vi "Configure Trigger.vi"(6 "Validation Channel (0: A)":i32(ring) items=["A", "B", "A/B"], 7 "Trigger Mode (0: mttAuto)":i32(ring) items=["mttAuto", "mttTrigger", "mttValLoose", "mttValNorm", "mttValTight"], 8 "error in (no error)":errorcluster, 9 "Trigger Delay (0 s)":dbl, 10 "Analyzer (0: A0)":i32(ring) items=["A0", "A1"], 11 "VISA resource name":refnum<visa-resource-name>) -> (0 "error out":errorcluster, 3 "VISA resource name out":refnum<visa-resource-name>)   [LabVIEW 2014, in "Stanford Research SR1.lvlib"]
doc: "Configures the attributes for the Trigger."
uses:
  Stanford Research SR1.lvlib
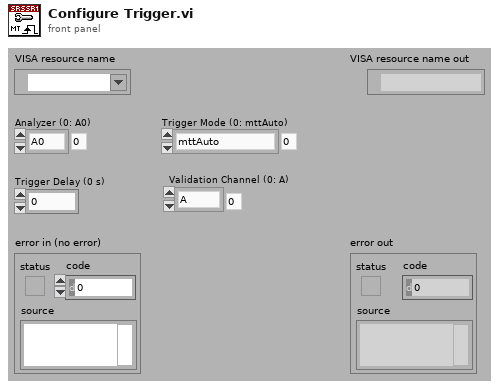
[diagram p1: front panel]
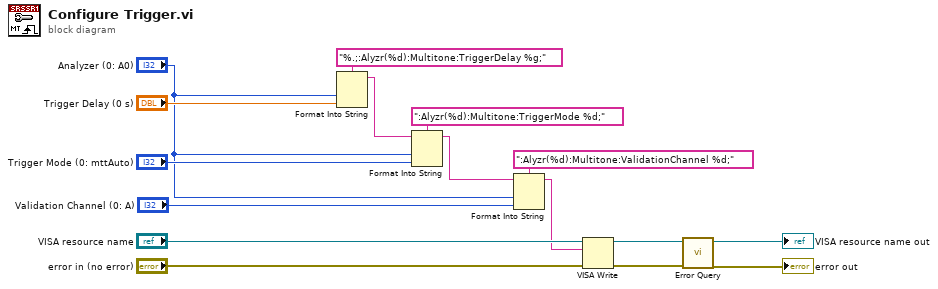
[diagram p0: block diagram]
diagram:
  n1 = Format Into String(format string="%.;:Alyzr(%d):Multitone:TriggerDelay %g;", "Analyzer (0: A0)", "Trigger Delay (0 s)") -> (resulting string=w15:string)  [unwired: 2 in, 1 out]
  n2 = Format Into String(format string=":Alyzr(%d):Multitone:TriggerMode %d;", initial string=w15, "Analyzer (0: A0)", "Trigger Mode (0: mttAuto)") -> (resulting string=w4:string)  [unwired: 1 in, 1 out]
  n3 = Format Into String(format string=":Alyzr(%d):Multitone:ValidationChannel %d;", initial string=w4, "Analyzer (0: A0)", "Validation Channel (0: A)") -> (resulting string=w1:string)  [unwired: 1 in, 1 out]
  n4 = VISA Write(VISA resource name="VISA resource name", write buffer=w1, error in (no error)="error in (no error)") -> (VISA resource name out=w11:refnum<visa-resource-name>, error out=w10:errorcluster)  [unwired: 1 out]
  n5 = call "Error Query.vi"("error in (no error)"=w10, "VISA resource name"=w11) -> ("error out"=→"error out":errorcluster, "VISA resource name out"=→"VISA resource name out":refnum<visa-resource-name>)  [unwired: 6 in, 2 out]
